vi "Real Compact Cho Inverse Matrix.vi"(0 "Compact Array":cluster{"Compact Array":dbl[], "array type":i32} {"array type" items=["lower triangular", "upper triangular", "symmetric matrix"]; "Compact Array" format="%.2f"}) -> (1 "Inverse Compact Array":cluster{"Compact Array":dbl[], "array type":i32} {"array type" items=["lower triangular", "upper triangular", "symmetric matrix"]; "Compact Array" format="%.2f"}, 2 "error":i32)   [LabVIEW 2017, in "NI_AALBase.lvlib"]
doc: "Finds the inverse matrix of the input matrix if it exists. If the input matrix is nonsingular, then the inverse matrix can be found by solving the linear system\n\n A B = I\n\n where\n A is the Input Matrix\n B is the Inverse Matrix\n I is the identity matirx."
uses:
  NI_AALBase.lvlib
  <resource>/lvanlys.dll
panel:
  # "Real Compact Cho Inverse Matrix"
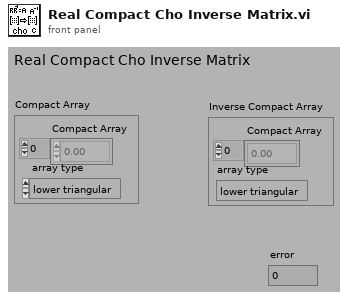
[diagram p1: front panel]
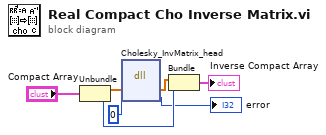
[diagram p0: block diagram]
diagram:
  n1 = Unbundle("Compact Array") -> ("Compact Array"=w6:dbl[], "array type"=w4:i32)
  n2 = dll-call lib="C:/Program Files (x86)/National Instruments/LabVIEW 2017/resource/lvanlys.*" fn="Cholesky_InvMatrix_head"("Compact Array"=w6, 0) -> ("Compact Array"=w5:dbl[], →"error":i32)  [unwired: 4 in, 2 out]
  n3 = Bundle("Compact Array"=w5, "array type"=w4) -> (→"Inverse Compact Array":cluster{"Compact Array":dbl[], "array type":i32})  [unwired: 1 in]
